vi "01 Washer HCC SM.vi"() -> ()   [LabVIEW 2011]
uses:
  HCC Data.ctl
  Washer Status Ctrl.ctl
  HCC Global Cluster Type.ctl
  <vilib>/Platform/fileVersionInfo.llb/FileVersionInformation.ctl
  GEA2 Washer Interface Ctrl.ctl
  Globals HCC.vi
panel:
  in  "Run":u32(colorbox)=6618880
  in  "Caution":u32(colorbox)=16776960
  in  "Uncofigured":u32(colorbox)=7171459
  in  "Configured":u32(colorbox)=16860
  in  "No Com":u32(colorbox)
  out "Row C":T1[](array[typedef])
  out "Init Com port message":string
  out "Row B":T1[](array[typedef])
  out "Row F":T1[](array[typedef])
  out "Row E":T1[](array[typedef])
  out "Row D":T1[](array[typedef])
  in  "Tab Control":T3(tab)=enum."View Streaming Data"
  out "Label Com Array":string[][](array[string])=[["M1", "100"], ["M3", "3"], ["M5", "5"], ["M7", "7"], ["M9", "9"], ["M11", "11"], ["M13", "13"], ["M15", "15"], ["M17", "17"], ["M19", "19"], ["M2", "2"], ["M4", "4"], ["M6", "6"], ["M8", "8"], ["M10", "10"], ["M12", "12"], ["M14", "14"], ["M16", "16"], ["M18", "18"], ["M20", "20"], ["N6", "21"], ["N7", "22"], ["N8", "23"], ["N9", "24"], ["N10", "25"], ["N11", "26"], ["N12", "27"], ["N13", "28"]]
  out "Current Filename":path
  in  "Config File":path=path "C:/Program Files/GE/Washer Hcc/HCC_Config.ini"
  out "Test Config Out":T4={"Directories"={"Com Port Config Filename"=path "D:/Work/HCC_Config.csv", "Save File Directory"=path "D:/Data", "Library Batch File"=path "c:/Data"}, "Test Information"={"Timeout"=1000, "Data Set ID"="HCC Rows A-D"}}
  in  "Timeout":i32=1000
  out "Save File Path":path=path "C:/Data"
  out "FileVersionInfo Out":T5
  out "Debug State Array":string[](array[string])
  out "Saving":errorcluster
  out "Log Coms Array":string[](array[string])
  out "Data Present":bool[](array[boolean])
  out "Partial Messages Out":cluster{"Partial Message Out":u8[]}[](array[cluster])
  in  "Select Station":string(combo)
  in  "Debug Log":string
  in  "Row Size Limits":i32[](array[numeric])=[9, 14, 19, 14, 20, 11]
  in  "Init":bool
  out "Read_ACK":bool
  out "Reading":bool
  in  "Row A":T1[](array[typedef])
  in  "Exit":bool
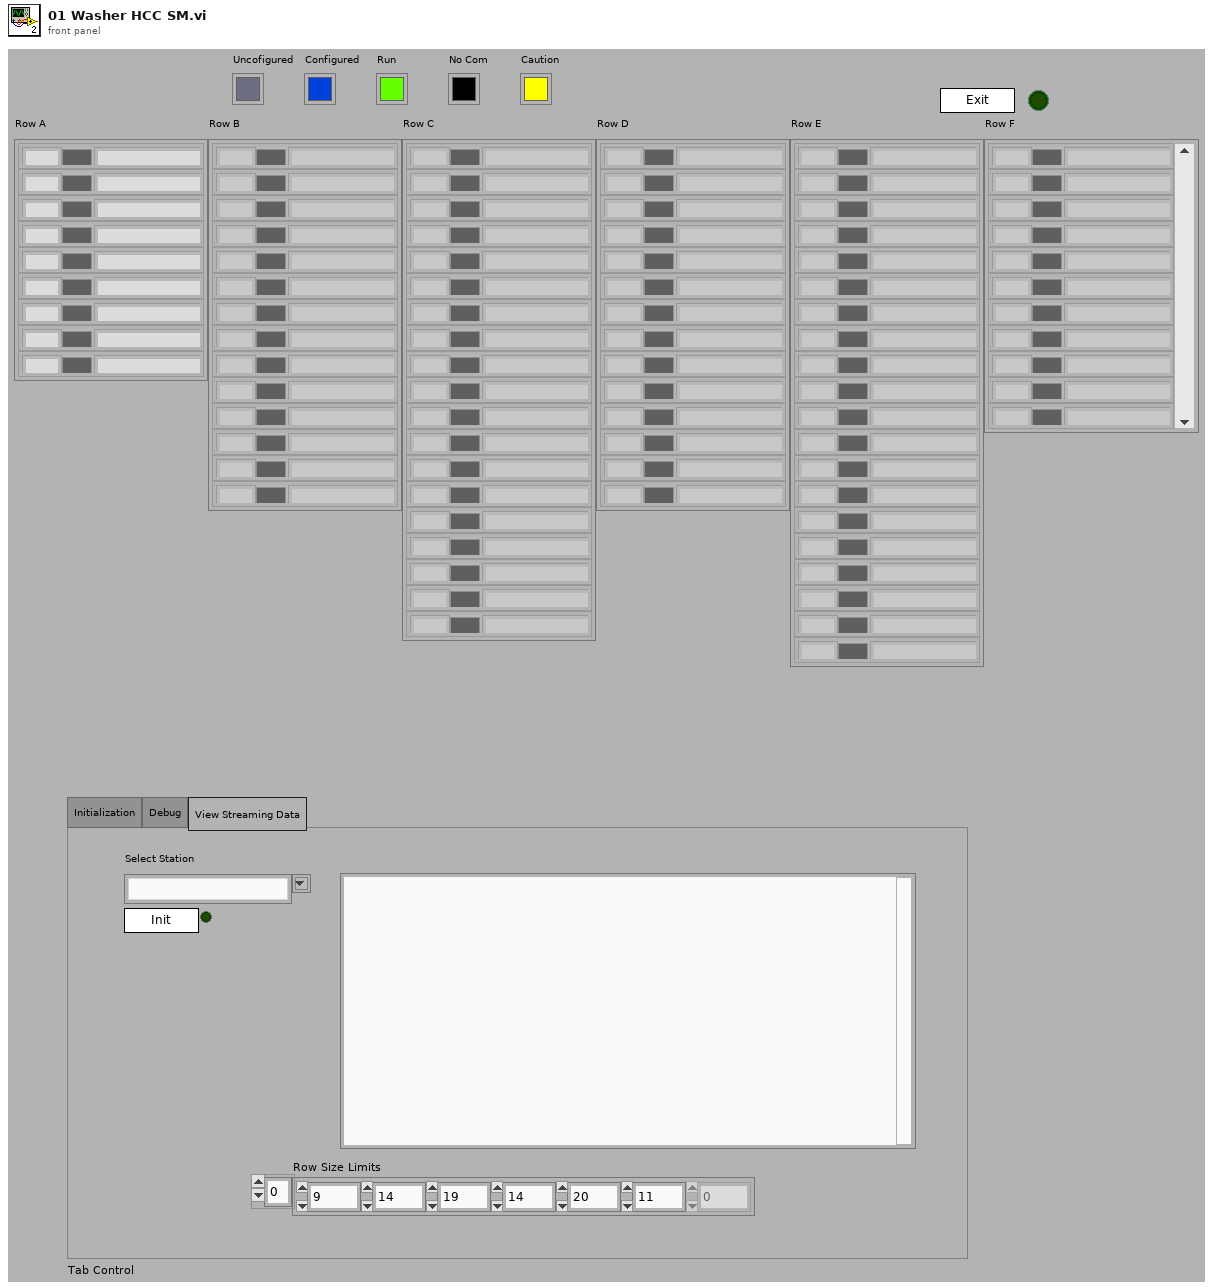
[diagram p1: front panel]
types:
  T1 = typedef "HCC Data.ctl" = cluster{"Station":string, "Color":u32, "Status":T2, "Error Time":string, "Com Err Count":u32, "Debug Log":string}
  T2 = typedef "Washer Status Ctrl.ctl" = enum16{"Running", "Err", "No Com", "No Conf"}
  T3 = enum32{"Initialization", "Debug", "View Streaming Data"}
  T4 = typedef "HCC Global Cluster Type.ctl" = cluster{"Directories":cluster{"Com Port Config Filename":path, "Save File Directory":path, "Library Batch File":path}, "Test Information":cluster{"Timeout":i32, "Data Set ID":string}}
  T5 = typedef "FileVersionInformation.ctl" = cluster{"FileVersion":string, "ProductName":string, "InternalName":string, "CompanyName":string, "LegalCopyright":string, "FileDescription":string}
  T6 = typedef "GEA2 Washer Interface Ctrl.ctl" = enum16{"Init Com Port", "SendCMD", "ReadPort", "Close Port", "Send Byte Data", "Read Continuous"}
  T7 = enum32{"invalid app kind", "Development System", "Run Time System", "Student Edition", "Embedded LabVIEW", "Evaluation", "Custom"}
  T8 = enum32{"Invalid", "Standard", "Closed", "Hidden", "Minimized", "Maximized"}
  T9 = cluster{"Core":cluster{"Current VI Reference":refnum<vi>, "Close Panel on Exit?":bool}, "Label Com Array":string[][], "Row A":T1[], "Com Array":u8[], "Save File Directory":path, "Last Hour":string, "Library Batch File":path, "Data Set ID":string}
  T10 = cluster{"Current VI Reference":refnum<vi>, "Close Panel on Exit?":bool}
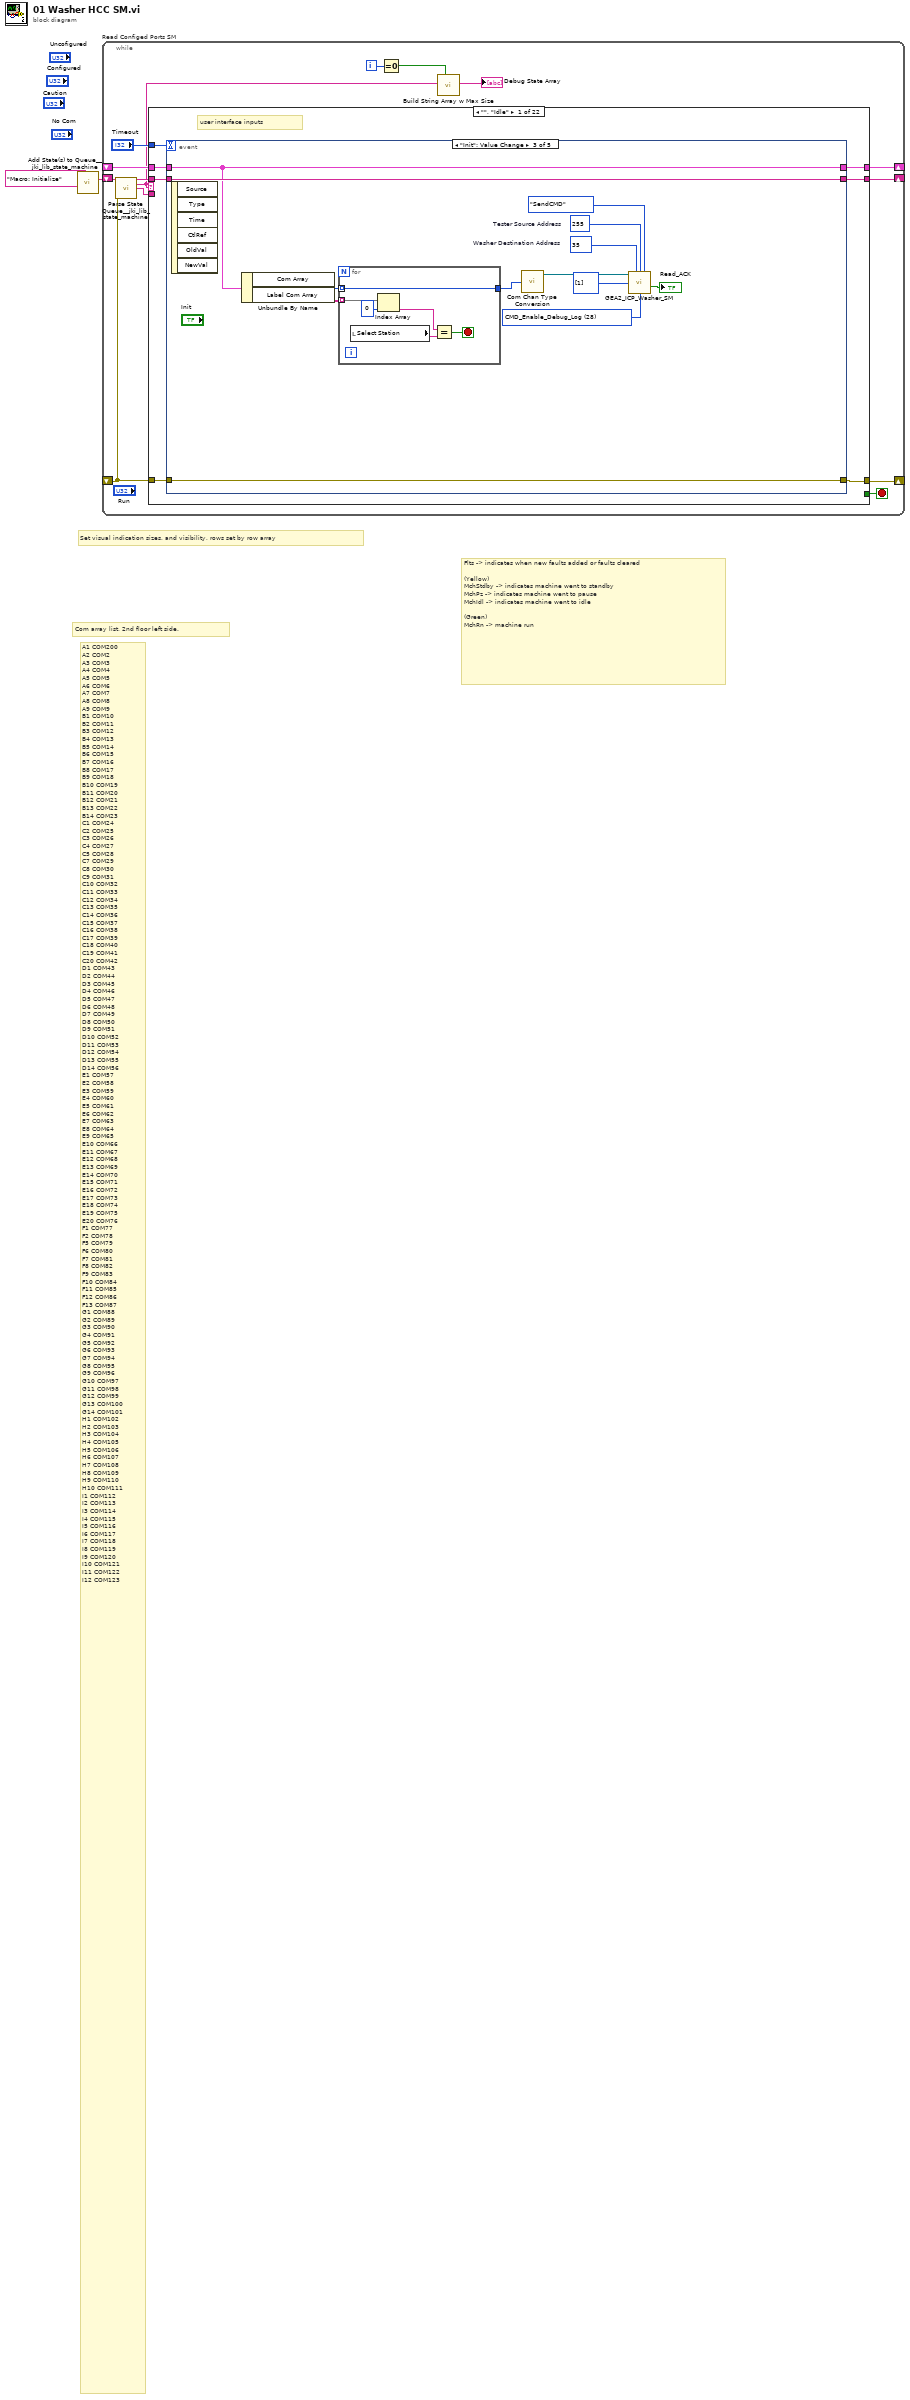
[diagram p0: block diagram]
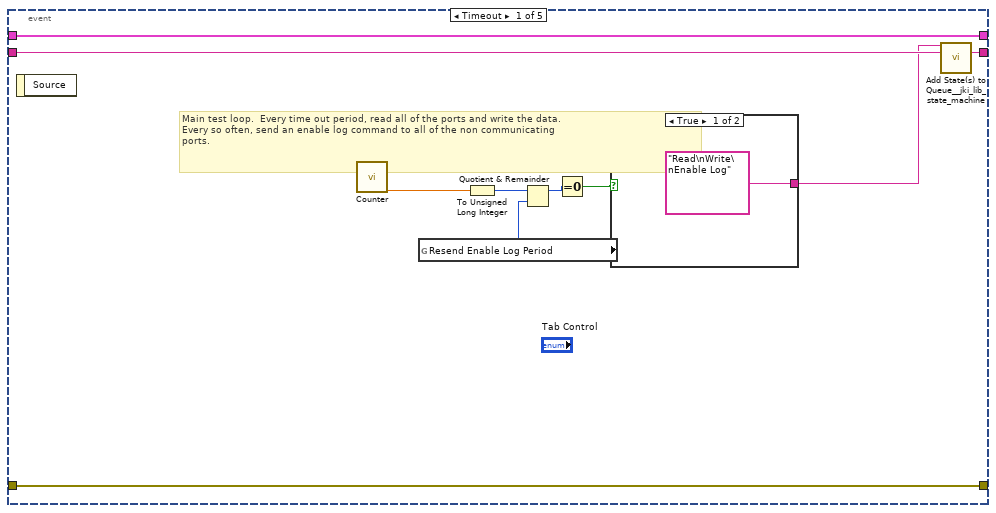
[diagram p2: hidden frame]
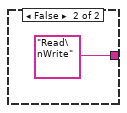
[diagram p3: hidden frame]
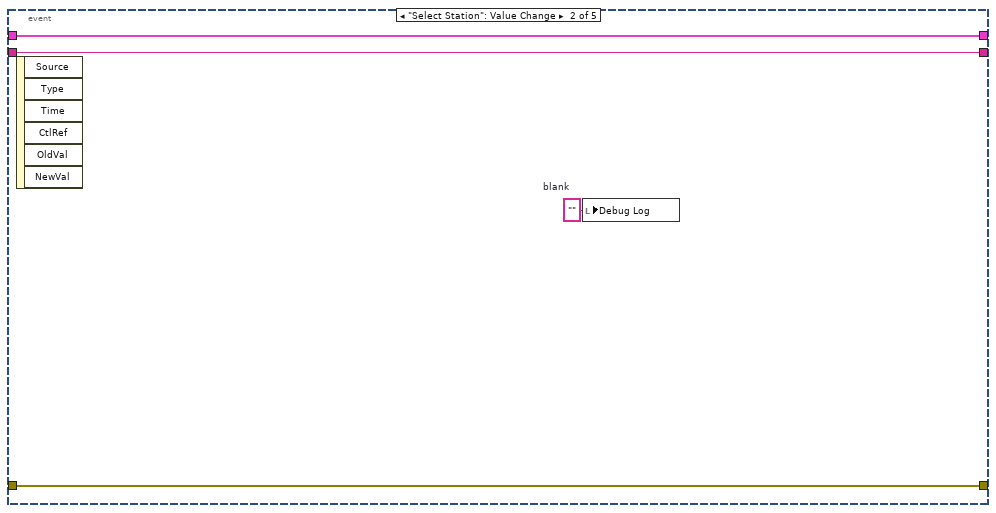
[diagram p4: hidden frame]
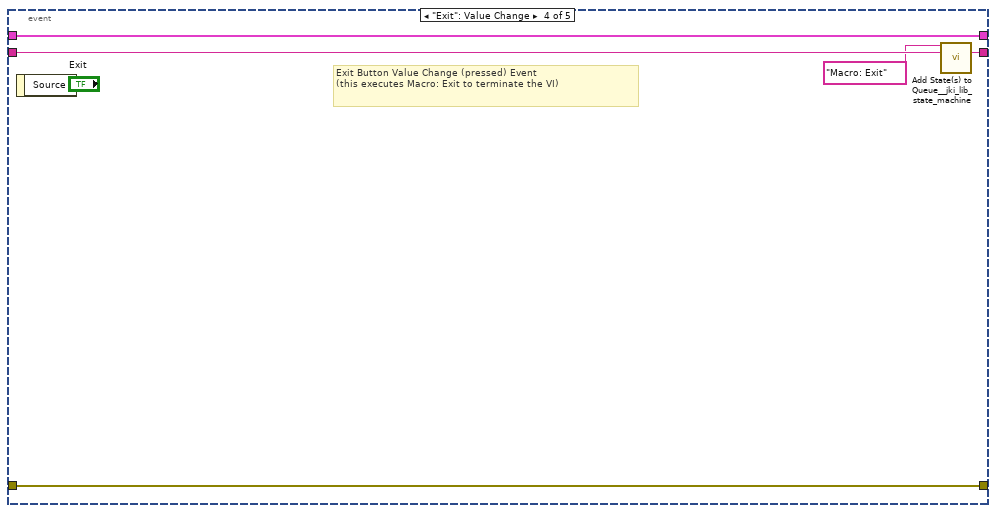
[diagram p5: hidden frame]
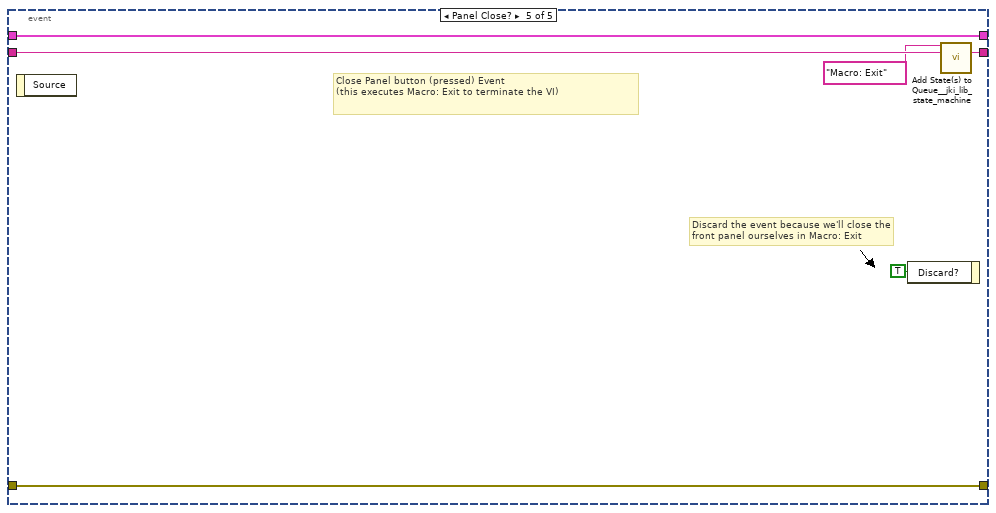
[diagram p6: hidden frame]
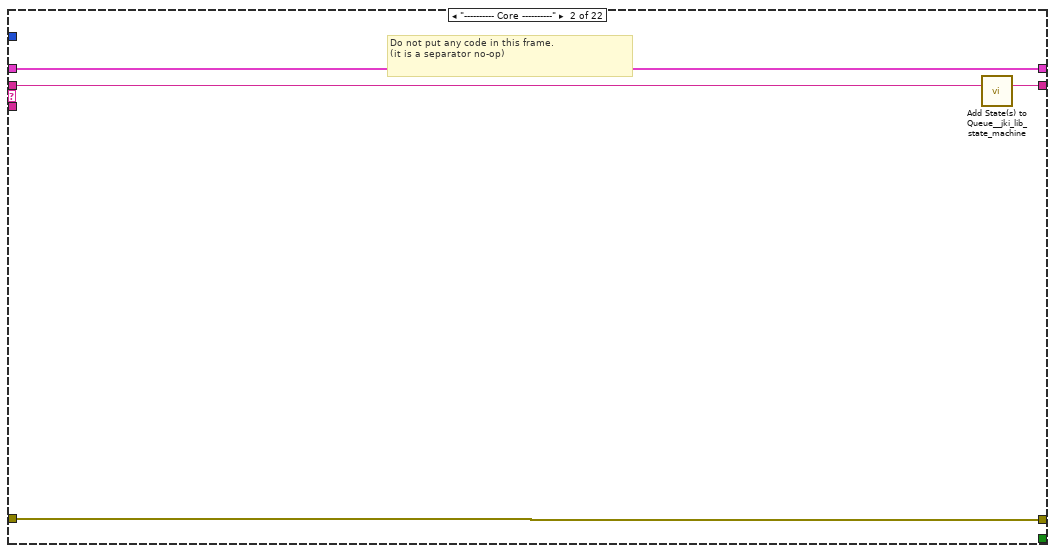
[diagram p7: hidden frame]
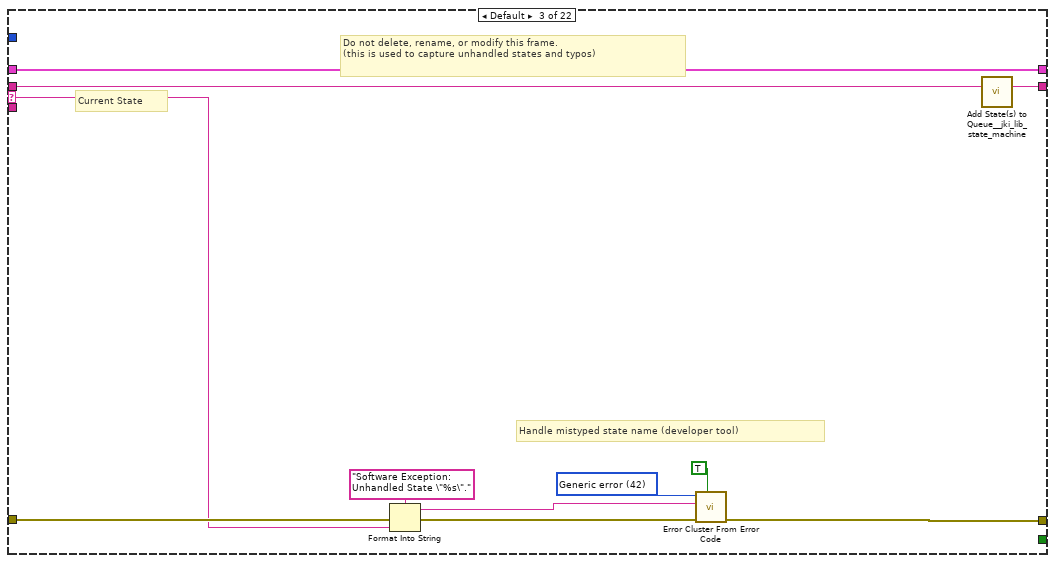
[diagram p8: hidden frame]
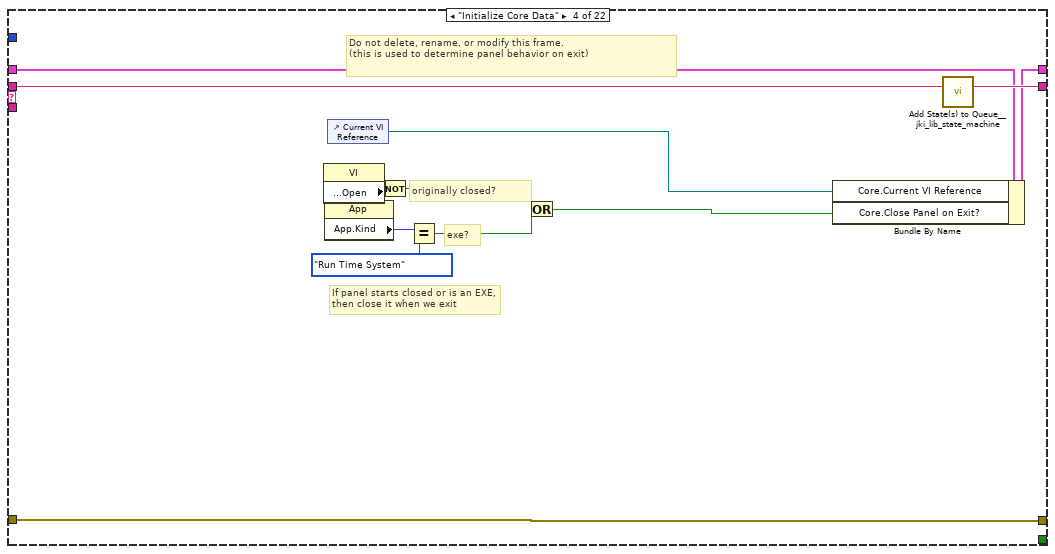
[diagram p9: hidden frame]
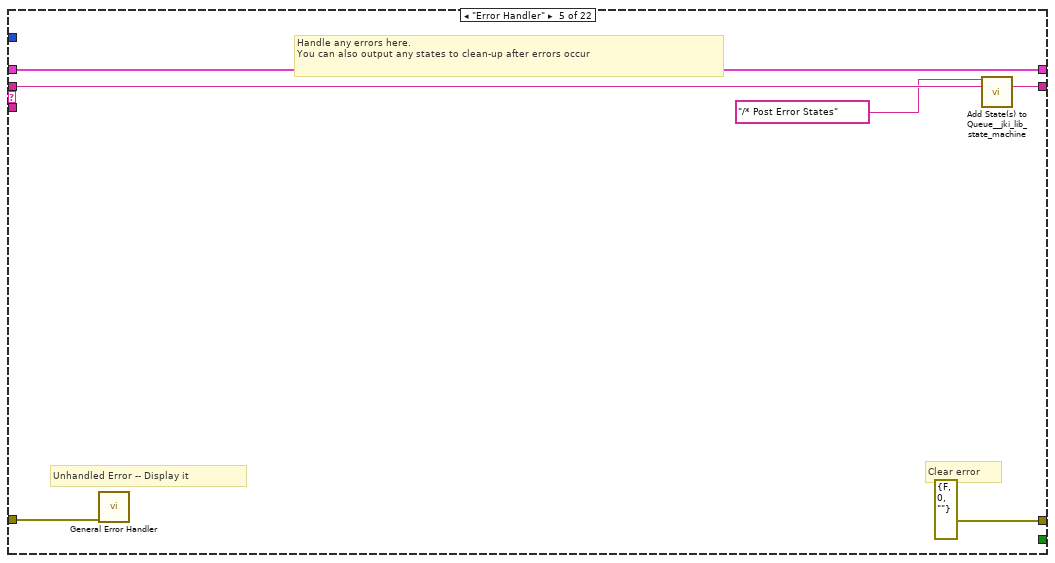
[diagram p10: hidden frame]
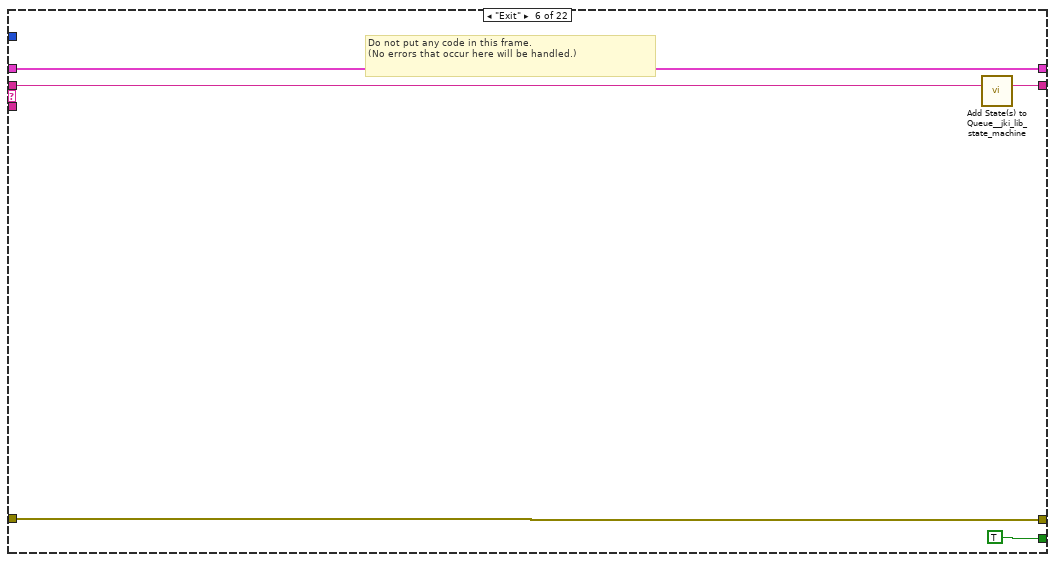
[diagram p11: hidden frame]
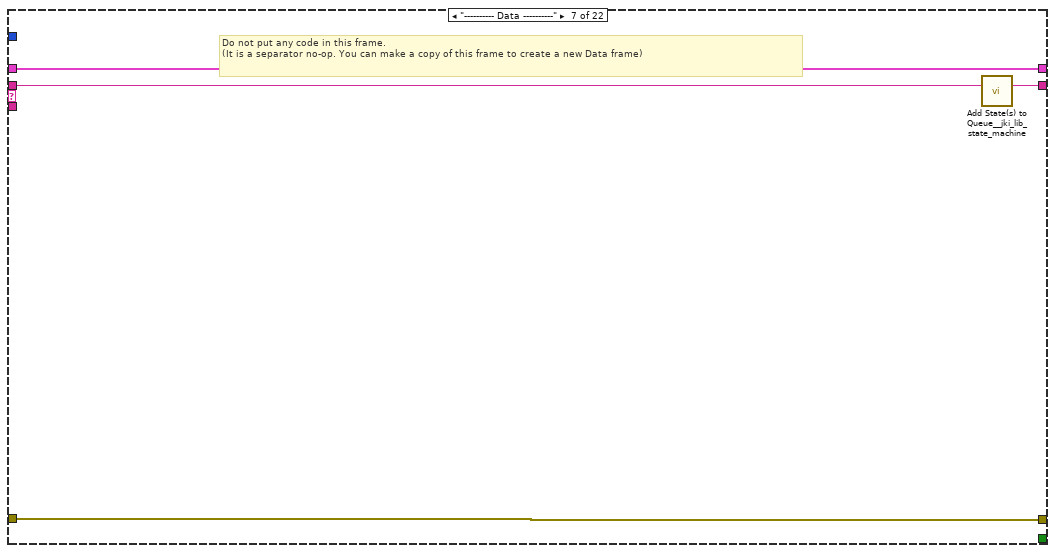
[diagram p12: hidden frame]
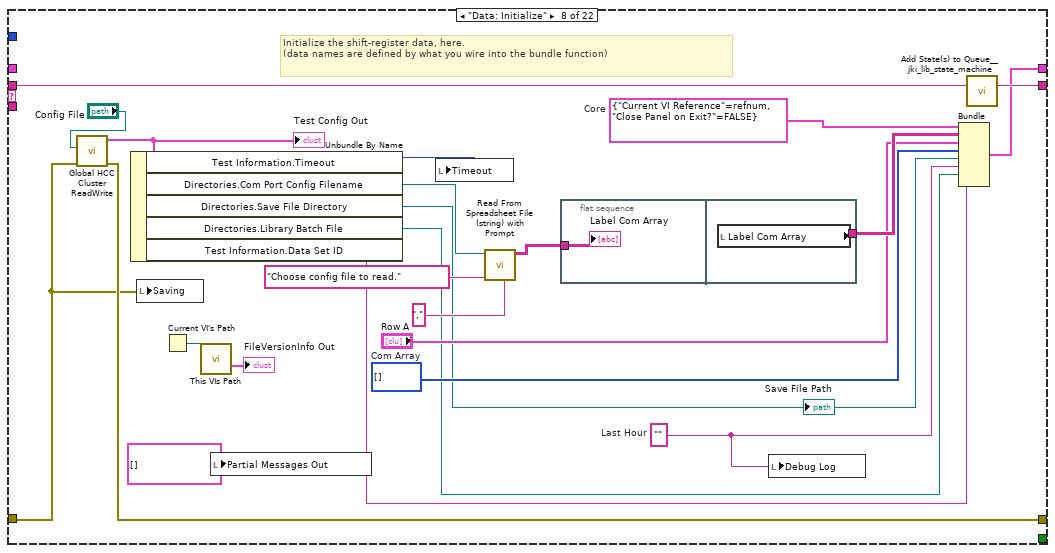
[diagram p13: hidden frame]
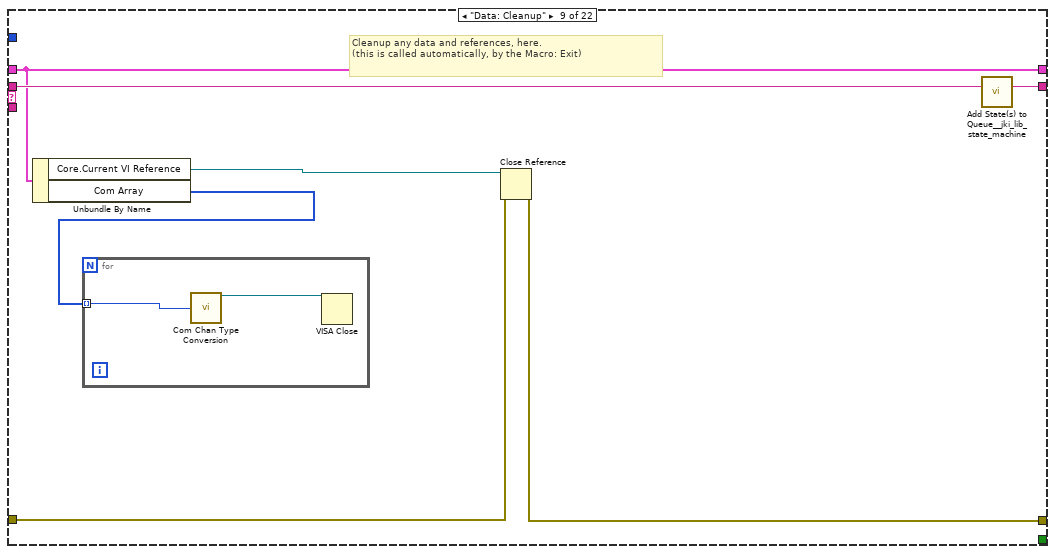
[diagram p14: hidden frame]
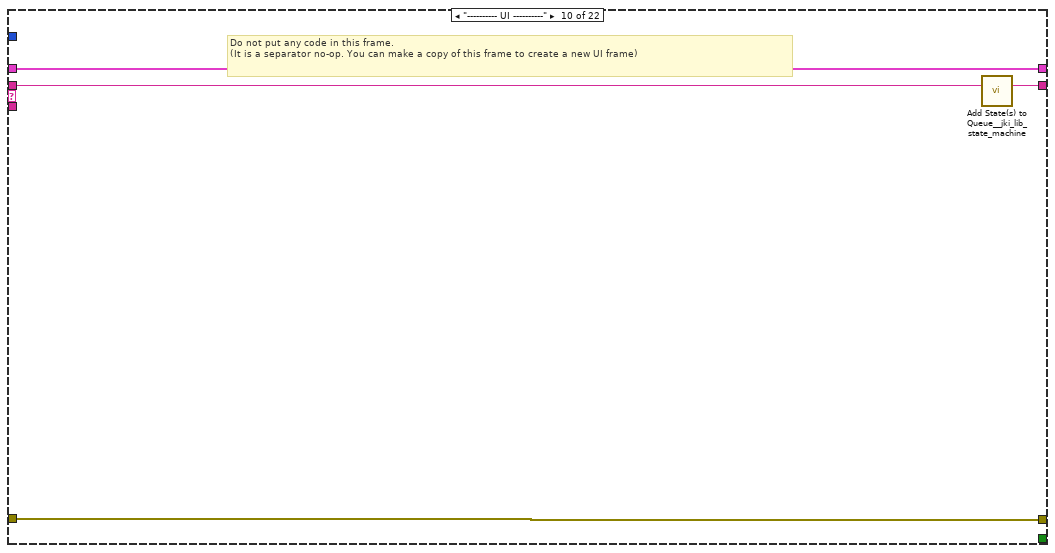
[diagram p15: hidden frame]
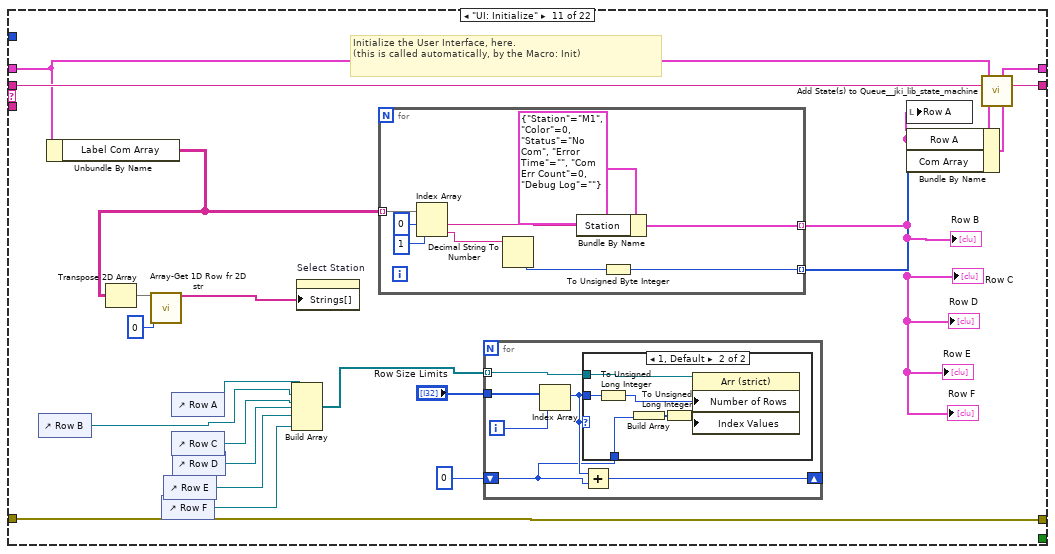
[diagram p16: hidden frame]
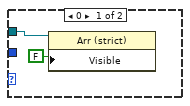
[diagram p17: hidden frame]
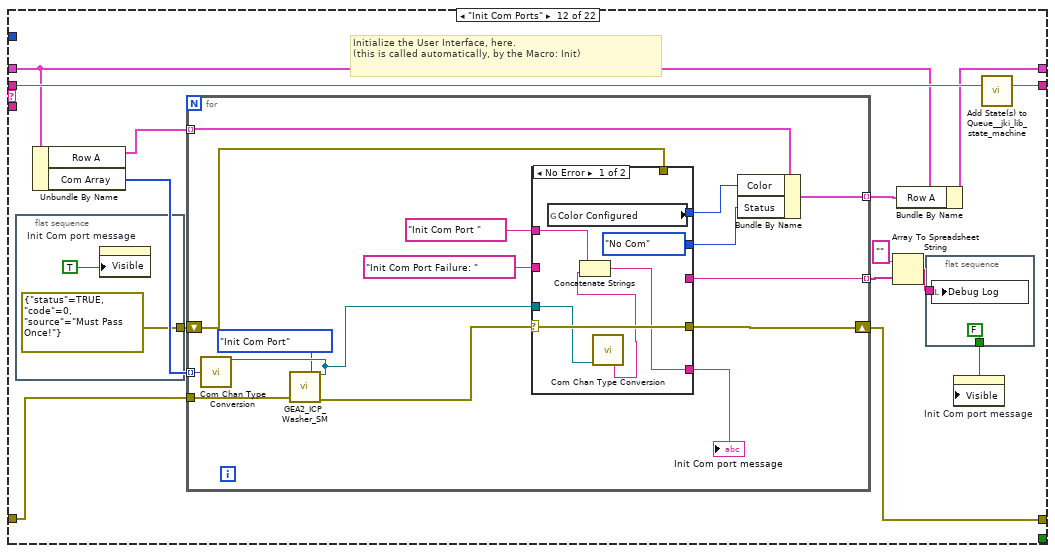
[diagram p18: hidden frame]
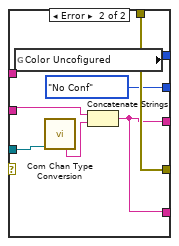
[diagram p19: hidden frame]
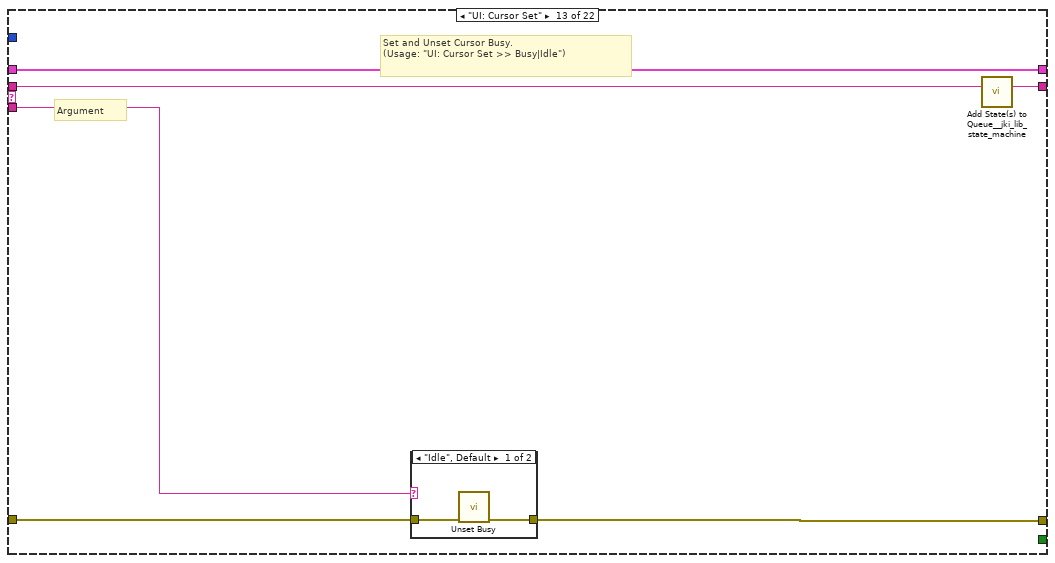
[diagram p20: hidden frame]
diagram:
  # "Com array list, 2nd floor left side."
  # "A1\tCOM200\nA2\tCOM2\nA3\tCOM3\nA4\tCOM4\nA5\tCOM5\nA6\tCOM6\nA7\tCOM7\nA8\tCOM8\nA9\tCOM9\nB1\tCOM10\nB2\tCOM11\nB3\tCOM12\nB4\tCOM13\nB5\tCOM14\nB6\tCOM15\nB7\tCOM16\nB8\tCOM17\nB9\tCOM18\nB10\tCOM19\nB11\tCOM20\nB12\tCOM21\nB13\tCOM22\nB14\tCOM23\nC1\tCOM24\nC2\tCOM25\nC3\tCOM26\nC4\tCOM27\nC5\tCOM28\nC7\tCOM29\nC8\tCOM30\nC9\tCOM31\nC10\tCOM32\nC11\tCOM33\nC12\tCOM34\nC13\tCOM35\nC14\tCOM36\nC15\tCOM37\nC16\tCOM38\nC17\tCOM39\nC18\tCOM40\nC19\tCOM41\nC20\tCOM42\nD1\tCOM43\nD2\tCOM44\nD3\tCOM45\nD4\tCOM46\nD5\tCOM47\nD6\tCOM48\nD7\tCOM49\nD8\tCOM50\nD9\tCOM51\nD10\tCOM52\nD11\tCOM53\nD12\tCOM54\nD13\tCOM55\nD14\tCOM56\nE1\tCOM57\nE2\tCOM58\nE3\tCOM59\nE4\tCOM60\nE5\tCOM61\nE6\tCOM62\nE7\tCOM63\nE8\tCOM64\nE9\tCOM65\nE10\tCOM66\nE11\tCOM67\nE12\tCOM68\nE13\tCOM69\nE14\tCOM70\nE15\tCOM71\nE16\tCOM72\nE17\tCOM73\nE18\tCOM74\nE19\tCOM75\nE20\tCOM76\nF1\tCOM77\nF2\tCOM78\nF5\tCOM79\nF6\tCOM80\nF7\tCOM81\nF8\tCOM82\nF9\tCOM83\nF10\tCOM84\nF11\tCOM85\nF12\tCOM86\nF13\tCOM87\nG1\tCOM88\nG2\tCOM89\nG3\tCOM90\nG4\tCOM91\nG5\tCOM92\nG6\tCOM93\nG7\tCOM94\nG8\tCOM95\nG9\tCOM96\nG10\tCOM97\nG11\tCOM98\nG12\tCOM99\nG13\tCOM100\nG14\tCOM101\nH1\tCOM102\nH2\tCOM103\nH3\tCOM104\nH4\tCOM105\nH5\tCOM106\nH6\tCOM107\nH7\tCOM108\nH8\tCOM109\nH9\tCOM110\nH10\tCOM111\nI1\tCOM112\nI2\tCOM113\nI3\tCOM114\nI4\tCOM115\nI5\tCOM116\nI6\tCOM117\nI7\tCOM118\nI8\tCOM119\nI9\tCOM120\nI10\tCOM121\nI11\tCOM122\nI12\tCOM123"
  # "Set visual indication sizes, and visibility, rows set by row array"
  # "Flts -> indicates when new faults added or faults cleared\n\n(Yellow)\nMchStdby -> indicates machine went to standby\nMchPz -> indicates machine went to pause\nMchIdl -> indicates machine went to idle \n\n(Green)\nMchRn -> machine run"
  n1 = call <vilib>:"Add State(s) to Queue__jki_lib_state_machine.vi"("State(s) in (\"\")"="Macro: Initialize") -> ("States Out"=w2:string)  [unwired: 14 in]
  n2 = while "Read Configed Ports SM" {
    shift-right: [w10] -> _
    shift-left: _ -> [w9]
    shift-right: [w13] -> _
    shift-left: _ -> [w7]
    shift-right: [w12] -> _
    shift-left: w2 -> [w14]
    i -> [w3]
    stop <- w11 stop-if-true
    n3 = call <vilib>:"Parse State Queue__jki_lib_state_machine.vi"("State Queue"=w14, "Error In (no error)"=w7) -> ("Remaining States"=w16:string, "Current State"=w6:string, "Arguments"=w15:string)  [unwired: 11 in]
    n4 = case shown="\"\", \"Idle\"" w6 {
      selector: w6 -> [_ _ w74 _ _ _ _ _ _ _ _ _ _ _ _ _ _ _ _ _ _ _]
      tunnel: w16 -> [w23 w73 w78 w96 w102 w107 w111 w134 w143 w149 w169 w206 w245 w256 w282 w287 w297 w301 w314 w331 w369 w382]
      tunnel: w15 -> [_ _ _ _ _ _ _ _ _ _ _ _ w240 w250 _ _ _ _ _ _ _ _]
      tunnel: w9 -> [w21 w70 w76 w87 w99 w105 w108 _ w138 w146 w166 w198 w243 w252 w279 w284 w294 w298 w310 w328 w367 w378]
      tunnel: [w20 w71 w80 w93 errorcluster {"status"=FALSE, "code"=0, "source"=""} ("error out") w104 w109 w118 w139 w147 w167 w202 w241 w253 w280 w285 w295 w299 w312 w329 w357 w379] -> w13
      tunnel: w7 -> [w19 w71 w79 w93 w98 w104 w109 w112 w140 w147 w167 w203 w242 w254 w280 w285 w295 w299 w312 w329 w358 w380]
      tunnel: [w22 w72 w77 w95 w101 w106 w110 w133 w142 w148 w168 w205 w244 w255 w281 w286 w296 w300 w313 w330 w368 w381] -> w12
      tunnel: [_ _ _ _ _ TRUE _ _ _ _ _ _ _ _ _ _ _ _ _ _ _ _] -> w11
      tunnel: [w18 w70 w76 w94 w99 w105 w108 w132 w138 w146 w165 w197 w243 w252 w279 w284 w294 w298 w309 w328 w366 w378] -> w10
      tunnel: "Timeout" -> [w17 _ _ _ _ _ _ _ _ _ _ _ _ _ _ _ _ _ _ _ _ _]
      frame "", "Idle" {
        # "user interface inputs"
        n5 = event shown="[2] \"Init\": Value Change" {
          selector: _ -> [_ _ _ _ _]
          dyn-events: _ -> [_ _ _ _ _]
          timeout: w17 -> [_ _ _ _ _]
          tunnel: w23 -> [w33 w38 w52 w63 w69]
          tunnel: [w32 w38 w52 w62 w68] -> w22
          tunnel: w21 -> [w30 w37 w46 w60 w66]
          tunnel: [w31 w36 w51 w61 w67] -> w20
          tunnel: w19 -> [w31 w36 w51 w61 w67]
          tunnel: [w30 w37 w46 w60 w66] -> w18
          event Timeout {
            # "Main test loop.  Every time out period, read all of the ports and write the data.\nEvery so often, send an enable log command to all of the non communicating\nports."
            n6 = event-data() -> ()  [unwired: 1 in, 1 out]
            n7 = call "Counter.vi"() -> ("Count"=w28:dbl)  [unwired: 11 in]
            n8 = global read "Globals HCC.vi" "Resend Enable Log Period"() -> (w27:u32)
            n9 = To Unsigned Long Integer(number=w28) -> (unsigned 32bit integer=w24:u32)
            n10 = Quotient & Remainder(x=w24, y=w27) -> (x-y*floor(x/y)=w26:u32)  [unwired: 1 out]
            n11 = Equal To 0?(x=w26) -> (x = 0?=w25:bool)
            n12 = case shown="True" w25 {
              tunnel: ["Read\nWrite\nEnable Log" ("State(s) in Front (\"\")") "Read\nWrite" ("State(s) in Front (\"\")")] -> w29
              frame True {
              }
              frame False {
              }
            }
            n13 = call <vilib>:"Add State(s) to Queue__jki_lib_state_machine.vi"("State(s) in Front (\"\")"=w29, "State(s) in (\"\")"=w33) -> ("States Out"=w32:string)  [unwired: 13 in]
          }
          event "Select Station": Value Change {
            w39 = ""  # blank
            n14 = event-data() -> ()  [unwired: 1 in, 6 out]
            n15 = local write "Debug Log"(w39) -> ()
          }
          event "Init": Value Change {
            w41 = u8 28 items=["CMD_Entry_Command", "CMD_Load_Control", "RQST_Input_Status", "CMD_LED_Control", "RQST_Encoder_Position_Status", "RQST_A2D_Status", "RQST_Switch_States_Status", "CMD_Buzzer_Control", "CMD_Shift_to_Spin", "CMD_Shift_to_Agitate", "RQST_Mode_Shift_Complete_Status", "CMD_Control_Inverter", "CMD_Spin_Action", "CMD_Agitate_Action", "RQST_Total_Switch_Status", "RQST_Total_Encoder_Status", "CMD_Test_Eeprom", "RQST_Eeprom_Test_Status", "CMD_Power_Mode", "RQST_Error_Status", "RQST_Get_Version", "CMD_Set_Personality", "RQST_Get_Personality", "CMD_Serial_Number", "RQST_Serial_Number_Status", "CMD_Model_Number", "RQST_Model_Number_Status", "CMD_Enter_Boot_Loader", "CMD_Enable_Debug_Log"] ("Command")
            w49 = u8 255  # Tester Source Address
            w50 = u8 35  # Washer Destination Address
            n16 = event-data() -> ()  [unwired: 1 in, 6 out]
            n17 = Unbundle By Name(w46) -> ("Com Array"=w48:u8[], "Label Com Array"=w47:string[][])
            n18 = for {
              tunnel: w47 -> [w58] mode=indexing
              tunnel: w48 -> [w53] mode=indexing
              tunnel: [w53] -> w45
              stop <- w55 stop-if-true
              n19 = local read "Select Station"() -> (w54:string)
              n20 = Index Array(array=w58, index=0) -> (element=w56:string)
              n21 = Equal?(x=w56, y=w54) -> (x = y?=w55:bool)
            }
            n22 = call "Com Chan Type Conversion.vi"("Com Chan"=w45) -> ("VISA resource name"=w44:refnum<visa-resource-name>)  [unwired: 11 in, 3 out]
            n23 = call "GEA2_ICP_Washer_SM.vi"("ComPort"=w44, "Destination Address"=w50, "Source Address"=w49, "Mode"=GEA2_Washer_Interface_Ctrl."SendCMD", "Byte Data"=u8[] [1], "Command"=w41) -> ("WriteOK"=→"Read_ACK":bool)  [unwired: 6 in, 3 out]
          }
          event "Exit": Value Change {
            # "Exit Button Value Change (pressed) Event\n(this executes Macro: Exit to terminate the VI)"
            n24 = event-data() -> ()  [unwired: 1 in, 1 out]
            n25 = call <vilib>:"Add State(s) to Queue__jki_lib_state_machine.vi"("State(s) in Front (\"\")"="Macro: Exit", "State(s) in (\"\")"=w63) -> ("States Out"=w62:string)  [unwired: 13 in]
          }
          event Panel Close? {
            # "Discard the event because we'll close the front panel ourselves in Macro: Exit"
            # "Close Panel button (pressed) Event\n(this executes Macro: Exit to terminate the VI)"
            n26 = event-data() -> ()  [unwired: 1 in, 1 out]
            n27 = event-data("Discard?"=TRUE) -> ()  [unwired: 1 in, 1 out]
            n28 = call <vilib>:"Add State(s) to Queue__jki_lib_state_machine.vi"("State(s) in Front (\"\")"="Macro: Exit", "State(s) in (\"\")"=w69) -> ("States Out"=w68:string)  [unwired: 13 in]
          }
        }
      }
      frame "---------- Core ----------" {
        # "Do not put any code in this frame.\n(it is a separator no-op)"
        n29 = call <vilib>:"Add State(s) to Queue__jki_lib_state_machine.vi"("State(s) in (\"\")"=w73) -> ("States Out"=w72:string)  [unwired: 14 in]
      }
      frame Default {
        w83 = 42 items=["No error", "Argument error", "Memory is full", "Out of zone", "End of file", "File already open", "Generic file I/O error", "File not found", "File permission error", "Disk is full", "Duplicate path", "Too many files open", "System feature not enabled", "Resource file not found", "Cannot add resource", "Resource not found", "Image not found", "Image memory error", "Pen does not exist", "Config type invalid", "Config token not found", "Config parse error", "Config memory error", "Bad external code format", "Bad external code offset", "External code not present", "Null window", "Destroy window error", "Null menu", "Print aborted", "Bad print record", "Print driver error", "Windows error during printing", "Memory error during printing", "Print dialog error", "Generic print error", "Invalid device refnum", "Device not found", "Device parameter error", "Device unit error", "Cannot open device", "Device call aborted", "Generic error", "Cancelled by user", "Object ID too low", "Object ID too high", "Object not in heap", "Unknown heap", "Unknown object (invalid DefProc)", "Unknown object (DefProc not in table)", "Message out of range", "Invalid (null) method", "Unknown message", "Manager call not supported", "Bad address", "Network operation in progress", "Network operation timed out", "Connection is busy", "Network attribute not supported", "Network error", "Address in use", "System out of memory", "Connection aborted", "Connection refused", "Not connected", "Already connected", "Connection closed", "Initialization error (interapplication manager)", "Bad occurrence", "Wait on unbound occurrence handler", "Occurrence queue overflow", "Datalog type conflict", "Unused", "Unrecognized type (interapplication manager)", "Memory corrupt", "Failed to make temporary DLL", "Old CIN version", "Drag socket not found", "Failed to load drop-object", "Failed to register OLE object", "Failed to release OLE object", "Format specifier type mismatch", "Unknown format specifier", "Too few format specifiers", "Too many format specifiers", "Scan failed", "Newer CIN version", "Error converting to variant", "Runtime menu error", "Password tampered", "Variant attribute not found", "Incompatible variant data type", "Event data is not available", "Event Store is not present", "Occurrence is not found", "Event Queue is not created", "Event info is not available", "Refnum passed is NULL", "Error retrieving Class GUID", "Error retrieving CoClass GUID", "Error retrieving TypeLib GUID.", "Bad built application magic bytes.", "Specific driver is different from the specific driver associated with the Logical Name.", "There is no session opened to the class driver.", "Max Error", "MAX - Error with config objects", "MAX - Error loading configuration", "MAX - Group not supported"]
        # "Current State"
        # "Do not delete, rename, or modify this frame.\n(this is used to capture unhandled states and typos)"
        # "Handle mistyped state name (developer tool)"
        n30 = Format Into String(format string="Software Exception: Unhandled State \"%s\"." ("message"), error in=w79, w74) -> (resulting string=w82:string, error out=w81:errorcluster)  [unwired: 1 in]
        n31 = call <vilib>:"Error Cluster From Error Code.vi"("show call chain? (False)"=TRUE, "error in (no error)"=w81, "error message (\"\")"=w82, "error code (0)"=w83) -> ("error out"=w80:errorcluster)  [unwired: 5 in]
        n32 = call <vilib>:"Add State(s) to Queue__jki_lib_state_machine.vi"("State(s) in (\"\")"=w78) -> ("States Out"=w77:string)  [unwired: 14 in]
      }
      frame "Initialize Core Data" {
        # "Do not delete, rename, or modify this frame.\n(this is used to determine panel behavior on exit)"
        # "originally closed?"
        # "exe?"
        # "If panel starts closed or is an EXE, then close it when we exit"
        n33 = property class="VI"() -> ("Front Panel.Open"=w92:bool)  [unwired: 2 in, 2 out]
        n34 = property class="App"() -> ("App.Kind"=w91:T7)  [unwired: 2 in, 2 out]
        n35 = control-ref of="Current VI Reference"() -> (w85:refnum<vi>)
        n36 = Not(x=w92) -> (.not. x?=w89:bool)
        n37 = Equal?(x=w91, y=T7."Run Time System" ("Application:Kind")) -> (x = y?=w88:bool)
        n38 = Or(x=w89, y=w88) -> (x .or. y?=w86:bool)
        n39 = Bundle By Name(cluster=w87, "Core.Current VI Reference"=w85, "Core.Close Panel on Exit?"=w86) -> (w94:T9)
        n40 = call <vilib>:"Add State(s) to Queue__jki_lib_state_machine.vi"("State(s) in (\"\")"=w96) -> ("States Out"=w95:string)  [unwired: 14 in]
      }
      frame "Error Handler" {
        # "Unhandled Error -- Display it"
        # "Handle any errors here.\nYou can also output any states to clean-up after errors occur"
        # "Clear error"
        n41 = call <vilib>:"General Error Handler.vi"("error in (no error)"=w98) -> ()  [unwired: 10 in, 5 out]
        n42 = call <vilib>:"Add State(s) to Queue__jki_lib_state_machine.vi"("State(s) in Front (\"\")"="/* Post Error States", "State(s) in (\"\")"=w102) -> ("States Out"=w101:string)  [unwired: 13 in]
      }
      frame "Exit" {
        # "Do not put any code in this frame.\n(No errors that occur here will be handled.)"
        n43 = call <vilib>:"Add State(s) to Queue__jki_lib_state_machine.vi"("State(s) in (\"\")"=w107) -> ("States Out"=w106:string)  [unwired: 14 in]
      }
      frame "---------- Data ----------" {
        # "Do not put any code in this frame.\n(It is a separator no-op. You can make a copy of this frame to create a new Data frame)"
        n44 = call <vilib>:"Add State(s) to Queue__jki_lib_state_machine.vi"("State(s) in (\"\")"=w111) -> ("States Out"=w110:string)  [unwired: 14 in]
      }
      frame "Data: Initialize" {
        w124 = ""  # Last Hour
        w126 = u8[] []  # Com Array
        w131 = T10 {"Current VI Reference"=refnum, "Close Panel on Exit?"=FALSE}  # Core
        # "Initialize the shift-register data, here.\n(data names are defined by what you wire into the bundle function)"
        n45 = call "Global HCC Cluster ReadWrite.vi"("error in (no error)"=w112, "configuration file path"="Config File") -> ("error out"=w118:errorcluster, "Test Config Out"=w122:T4)  [unwired: 8 in]
        "Test Config Out" <- w122
        n46 = Unbundle By Name(w122) -> ("Test Information.Timeout"=w119:i32, "Directories.Com Port Config Filename"=w121:path, "Directories.Save File Directory"=w117:path, "Directories.Library Batch File"=w120:path, "Test Information.Data Set ID"=w116:string)
        "Save File Path" <- w117
        n47 = local write "Saving"(w112) -> ()
        n48 = Current VI's Path() -> (path=w114:path)
        n49 = call "This VIs Path.vi"("path"=w114) -> ("FileVersionInfo Out"=→"FileVersionInfo Out":T5)  [unwired: 10 in, 4 out]
        n50 = local write "Partial Messages Out"(cluster{"Partial Message Out":u8[]}[] [] ("Partial Messages Out")) -> ()
        n51 = local write "Timeout"(w119) -> ()
        n52 = call "Read From Spreadsheet File (string) with Prompt.vi"("delimiter (\\t)"="," ("delimiter (\\t)"), "prompt"="Choose config file to read.", "file path (dialog if empty)"=w121) -> ("all rows"=w129:string[][])  [unwired: 4 in, 4 out]
        n53 = flat-sequence {
          tunnel: w129 -> [w135]
          tunnel: [w136] -> w128
          frame #0 {
            "Label Com Array" <- w135
          }
          frame #1 {
            n54 = local read "Label Com Array"() -> (w136:string[][])
          }
        }
        n55 = local write "Debug Log"(w124) -> ()
        n56 = Bundle("Core"=w131, "Label Com Array"=w128, "Row A"="Row A", "Com Array"=w126, "Save File Directory"=w117, "Last Hour"=w124, "Library Batch File"=w120, "Data Set ID"=w116) -> (w132:T9)  [unwired: 1 in]
        n57 = call <vilib>:"Add State(s) to Queue__jki_lib_state_machine.vi"("State(s) in (\"\")"=w134) -> ("States Out"=w133:string)  [unwired: 14 in]
      }
      frame "Data: Cleanup" {
        # "Cleanup any data and references, here.\n(this is called automatically, by the Macro: Exit)"
        n58 = Unbundle By Name(w138) -> ("Core.Current VI Reference"=w141:refnum<vi>, "Com Array"=w137:u8[])
        n59 = for {
          tunnel: w137 -> [w145] mode=indexing
          n60 = call "Com Chan Type Conversion.vi"("Com Chan"=w145) -> ("VISA resource name"=w144:refnum<visa-resource-name>)  [unwired: 11 in, 3 out]
          n61 = VISA Close(VISA resource name=w144) -> ()  [unwired: 1 in, 1 out]
        }
        n62 = Close Reference(reference=w141, error in (no error)=w140) -> (error out=w139:errorcluster)
        n63 = call <vilib>:"Add State(s) to Queue__jki_lib_state_machine.vi"("State(s) in (\"\")"=w143) -> ("States Out"=w142:string)  [unwired: 14 in]
      }
      frame "---------- UI ----------" {
        # "Do not put any code in this frame.\n(It is a separator no-op. You can make a copy of this frame to create a new UI frame)"
        n64 = call <vilib>:"Add State(s) to Queue__jki_lib_state_machine.vi"("State(s) in (\"\")"=w149) -> ("States Out"=w148:string)  [unwired: 14 in]
      }
      frame "UI: Initialize" {
        # "Initialize the User Interface, here.\n(this is called automatically, by the Macro: Init)"
        n65 = control-ref of="Row B"() -> (w150:refnum<vi>)
        n66 = Unbundle By Name(w166) -> ("Label Com Array"=w162:string[][])
        n67 = Transpose 2D Array(2D array=w162) -> (transposed array=w163:string[][])
        n68 = call "Array-Get 1D Row fr 2D str.vi"("all rows"=w163, "row index"=0) -> ("row"=w160:string[])  [unwired: 13 in]
        n69 = control-ref of="Row F"() -> (w152:refnum<vi>)
        n70 = control-ref of="Row E"() -> (w155:refnum<vi>)
        n71 = control-ref of="Row A"() -> (w158:refnum<vi>)
        n72 = control-ref of="Row C"() -> (w157:refnum<vi>)
        n73 = control-ref of="Row D"() -> (w156:refnum<vi>)
        n74 = Build Array(w158, w150, w157, w156, w155, w152) -> (w154:refnum<vi>[])
        n75 = property on="Select Station" class="CmbBox"("Strings[]"=w160) -> ()  [unwired: 2 in, 2 out]
        n76 = for {
          tunnel: w162 -> [w192] mode=indexing
          tunnel: [w184] -> w164 mode=indexing
          tunnel: [w186] -> w151 mode=indexing
          n77 = Index Array(array=w192, index #1=0 ("index"), index #2=1 ("index")) -> (element #1=w188:string, element #2=w187:string)
          n78 = Decimal String To Number(string=w187) -> (number=w185:i32)  [unwired: 2 in, 1 out]
          n79 = Bundle By Name(cluster=T1 {"Station"="M1", "Color"=0, "Status"=enum."No Com", "Error Time"="", "Com Err Count"=0, "Debug Log"=""} ("Location:IND,Status,Message,No Com Count, Cycle Count"), "Station"=w188) -> (w186:T1)
          n80 = To Unsigned Byte Integer(number=w185) -> (unsigned 8bit integer=w184:u8)
        }
        "Row D" <- w151
        "Row E" <- w151
        "Row C" <- w151
        "Row F" <- w151
        "Row B" <- w151
        n81 = for {
          tunnel: w154 -> [w175] mode=indexing
          tunnel: "Row Size Limits" -> [w174]
          shift-right: [w171] -> _
          shift-left: 0 -> [w170]
          i -> [w173]
          n82 = Index Array(array=w174, index=w173) -> (element=w172:i32)
          n83 = case shown="1, Default" w172 {
            tunnel: w175 -> [w177 w183]
            tunnel: w172 -> [_ w182]
            tunnel: w170 -> [_ w178]
            frame 0 {
              n84 = property class="Arr (strict)"(reference=w177, "Visible"=FALSE) -> ()  [unwired: 1 in, 2 out]
            }
            frame 1, Default {
              n85 = To Unsigned Long Integer(number=w182) -> (unsigned 32bit integer=w181:u32)
              n86 = Build Array(w178) -> (w180:i32[])
              n87 = To Unsigned Long Integer(number=w180) -> (unsigned 32bit integer=w179:u32[])
              n88 = property class="Arr (strict)"(reference=w183, "Number of Rows"=w181, "Index Values"=w179) -> ()  [unwired: 1 in, 2 out]
            }
          }
          n89 = Add(x=w172, y=w170) -> (x+y=w171:i32)
        }
        n90 = local write "Row A"(w151) -> ()
        n91 = Bundle By Name(cluster=w166, "Row A"=w151, "Com Array"=w164) -> (w165:T9)
        n92 = call <vilib>:"Add State(s) to Queue__jki_lib_state_machine.vi"("State(s) in (\"\")"=w169) -> ("States Out"=w168:string)  [unwired: 14 in]
      }
      frame "Init Com Ports" {
        # "Initialize the User Interface, here.\n(this is called automatically, by the Macro: Init)"
        n93 = flat-sequence {
          tunnel: [errorcluster {"status"=TRUE, "code"=0, "source"="Must Pass Once!"} ("error IO")] -> w201
          frame #0 {
            n94 = property on="Init Com port message" class="Str"("Visible"=TRUE) -> ()  [unwired: 2 in, 2 out]
          }
        }
        n95 = Unbundle By Name(w198) -> ("Row A"=w200:T1[], "Com Array"=w204:u8[])
        n96 = for {
          tunnel: w204 -> [w224] mode=indexing
          tunnel: w203 -> [w225]
          shift-right: [w220] -> w202
          shift-left: w201 -> [w219]
          tunnel: w200 -> [w218] mode=indexing
          tunnel: [w216] -> w199 mode=indexing
          tunnel: [w215] -> w196 mode=indexing
          n97 = call "Com Chan Type Conversion.vi"("Com Chan"=w224) -> ("VISA resource name"=w223:refnum<visa-resource-name>)  [unwired: 11 in, 3 out]
          n98 = call "GEA2_ICP_Washer_SM.vi"("ComPort"=w223, "Mode"=GEA2_Washer_Interface_Ctrl."Init Com Port", "Error In"=w225) -> ("Error Out"=w222:errorcluster)  [unwired: 9 in, 3 out]
          n99 = case shown="No Error" w222 {
            selector: w222 -> [w232 _]
            tunnel: w223 -> [w228 w239]
            tunnel: "Init Com Port Failure: " -> [_ w238]
            tunnel: [w232 w236] -> w220
            tunnel: w219 -> [_ w236]
            tunnel: [w231 w235] -> w217
            tunnel: [_ w234] -> w215
            tunnel: "Init Com Port " -> [w230 _]
            tunnel: [w229 w234] -> w212
            tunnel: [Washer_Status_Ctrl."No Com" ("Status") Washer_Status_Ctrl."No Conf" ("Status")] -> w211
            frame No Error {
              n100 = global read "Globals HCC.vi" "Color Configured"() -> (w231:u32)
              n101 = call "Com Chan Type Conversion.vi"("Com Chan In"=w228) -> ("Com Text 2"=w227:string)  [unwired: 11 in, 3 out]
              n102 = Concatenate Strings(w230, w227) -> (w229:string)
            }
            frame Error {
              n103 = global read "Globals HCC.vi" "Color Uncofigured"() -> (w235:u32)
              n104 = call "Com Chan Type Conversion.vi"("Com Chan In"=w239) -> ("Com Text 2"=w237:string)  [unwired: 11 in, 3 out]
              n105 = Concatenate Strings(w238, w237) -> (w234:string)
            }
          }
          "Init Com port message" <- w212
          n106 = Bundle By Name(cluster=w218, "Color"=w217, "Status"=w211) -> (w216:T1)
        }
        n107 = Array To Spreadsheet String(array=w196, 3:"" ("format string")) -> (spreadsheet string=w195:string)  [unwired: 1 in]
        n108 = Bundle By Name(cluster=w198, "Row A"=w199) -> (w197:T9)
        n109 = flat-sequence {
          tunnel: w195 -> [w208]
          tunnel: [FALSE ("Visible")] -> w193
          frame #0 {
            n110 = local write "Debug Log"(w208) -> ()
          }
        }
        n111 = property on="Init Com port message" class="Str"("Visible"=w193) -> ()  [unwired: 2 in, 2 out]
        n112 = call <vilib>:"Add State(s) to Queue__jki_lib_state_machine.vi"("State(s) in (\"\")"=w206) -> ("States Out"=w205:string)  [unwired: 14 in]
      }
      frame "UI: Cursor Set" {
        # "Argument"
        # "Set and Unset Cursor Busy.\n(Usage: \"UI: Cursor Set >> Busy|Idle\")"
        n113 = case shown="\"Idle\", Default" w240 {
          tunnel: w242 -> [w247 w249]
          tunnel: [w246 w248] -> w241
          frame "Idle", Default {
            n114 = call <vilib>:"Unset Busy.vi"("error in (no error)"=w247) -> ("error out"=w246:errorcluster)  [unwired: 10 in]
          }
          frame "Busy" {
            n115 = call <vilib>:"Set Busy.vi"("error in (no error)"=w249) -> ("error out"=w248:errorcluster)  [unwired: 9 in, 1 out]
          }
        }
        n116 = call <vilib>:"Add State(s) to Queue__jki_lib_state_machine.vi"("State(s) in (\"\")"=w245) -> ("States Out"=w244:string)  [unwired: 14 in]
      }
      frame "UI: Front Panel State" {
        # "Argument"
        # "Set Front Panel Open or Closed\n(Usage: \"UI: Front Panel State >> Open|Close\")"
        n117 = Unbundle By Name(w252) -> ("Core.Current VI Reference"=w251:refnum<vi>)
        n118 = case shown="\"Open\", Default" w250 {
          tunnel: w254 -> [w260 w273]
          tunnel: [w262 w274] -> w253
          tunnel: w251 -> [w261 w271]
          frame "Open", Default {
            n119 = property class="VI"(reference=w261, error in=w260) -> (reference out=w258:refnum<vi>, error out=w259:errorcluster, "Front Panel.Open"=w257:bool)
            n120 = case shown="False" w257 {
              tunnel: [w265 w268] -> w262
              tunnel: w259 -> [w264 w268]
              tunnel: w258 -> [w263 _]
              frame False {
                n121 = invoke class="VI" method="FP.Open"(reference=w263, error in=w264, "Activate"=TRUE, "State"=T8."Standard") -> (error out=w265:errorcluster)  [unwired: 1 in, 4 out]
              }
              frame True {
              }
            }
          }
          frame "Close" {
            n122 = property class="VI"(reference=w271, error in=w273) -> (reference out=w270:refnum<vi>, error out=w272:errorcluster, "Front Panel.Open"=w269:bool)
            n123 = case shown="True" w269 {
              tunnel: [w275 w278] -> w274
              tunnel: w272 -> [w275 w277]
              tunnel: w270 -> [_ w276]
              frame False {
              }
              frame True {
                n124 = invoke class="VI" method="FP.Close"(reference=w276, error in=w277) -> (error out=w278:errorcluster)  [unwired: 1 in, 2 out]
              }
            }
          }
        }
        n125 = call <vilib>:"Add State(s) to Queue__jki_lib_state_machine.vi"("State(s) in (\"\")"=w256) -> ("States Out"=w255:string)  [unwired: 14 in]
      }
      frame "---------- Macro ----------" {
        # "Do not put any code in this frame.\n(It is a separator no-op. You can make a copy of this frame to create a new Macro frame)"
        n126 = call <vilib>:"Add State(s) to Queue__jki_lib_state_machine.vi"("State(s) in (\"\")"=w282) -> ("States Out"=w281:string)  [unwired: 14 in]
      }
      frame "Macro: Initialize" {
        w283 = "Data: Initialize\nInitialize Core Data\nUI: Initialize\nUI: Front Panel State >> Open\nInit Com Ports"  # Data: Initialize Initialize Core Data UI: Initialize UI: Front Panel State >> Open Init Com Ports
        # "Initialization Macro\n(This is called once, when the VI starts)"
        n127 = call <vilib>:"Add State(s) to Queue__jki_lib_state_machine.vi"("State(s) in Front (\"\")"=w283, "State(s) in (\"\")"=w287) -> ("States Out"=w286:string)  [unwired: 13 in]
      }
      frame "Macro: Exit" {
        # "Exit Macro\n(This is called once, when the VI exits)"
        n128 = Unbundle By Name(w294) -> ("Core.Close Panel on Exit?"=w293:bool)
        n129 = Select(t="UI: Front Panel State >> Close", s=w293, f="") -> (s? t:f=w290:string)
        n130 = call <vilib>:"Add State(s) to Queue__jki_lib_state_machine.vi"("State(s) in (\"\")"=w290, "State(s) at Back (\"\")"="Data: Cleanup\nExit") -> ("States Out"=w288:string)  [unwired: 13 in]
        n131 = call <vilib>:"Add State(s) to Queue__jki_lib_state_machine.vi"("State(s) in Front (\"\")"=w288, "State(s) in (\"\")"=w297) -> ("States Out"=w296:string)  [unwired: 13 in]
      }
      frame "---------- New Category ----------" {
        # "Template Separator\n(You can make a copy of, or modify, this frame)"
        n132 = call <vilib>:"Add State(s) to Queue__jki_lib_state_machine.vi"("State(s) in (\"\")"=w301) -> ("States Out"=w300:string)  [unwired: 14 in]
      }
      frame "Read" {
        # "read the serial ports"
        n133 = Unbundle By Name(w310) -> ("Com Array"=w311:u8[], "Row A"=w303:T1[])
        n134 = flat-sequence {
          tunnel: [w316] -> w304
          frame #0 {
            n135 = local read "Partial Messages Out"() -> (w316:cluster{"Partial Message Out":u8[]}[])
            n136 = local write "Reading"(TRUE ("Reading")) -> ()
          }
        }
        n137 = call "Read All Washers.vi"("Com Array"=w311, "HCC  Array In"=w303, "Partial Message Array"=w304) -> ("Log Coms Array"=→"Log Coms Array":string[], "HCC  Array Out"=w302:T1[], "Data Present"=→"Data Present":bool[], "Partial Messages Out"=→"Partial Messages Out":cluster{"Partial Message Out":u8[]}[])  [unwired: 8 in, 1 out]
        n138 = flat-sequence {
          tunnel: w302 -> [w318]
          frame #0 {
            n139 = local write "Row A"(w318) -> ()
            "Reading" <- FALSE ("Reading")
          }
        }
        n140 = Bundle By Name(cluster=w310, "Row A"=w302) -> (w309:T9)
        n141 = local write "Row C"(w302) -> ()
        n142 = local write "Row B"(w302) -> ()
        n143 = local write "Row D"(w302) -> ()
        n144 = local write "Row E"(w302) -> ()
        n145 = local write "Row F"(w302) -> ()
        n146 = call <vilib>:"Add State(s) to Queue__jki_lib_state_machine.vi"("State(s) in Front (\"\")"="Add Select Data" ("State(s) in Front (\"\")"), "State(s) in (\"\")"=w314) -> ("States Out"=w313:string)  [unwired: 13 in]
      }
      frame "Add Select Data" {
        # "Your code here.\n(You can make a copy of, or modify, this frame)"
        n147 = Unbundle By Name(w328) -> ("Label Com Array"=w327:string[][], "Row A"=w326:T1[])
        n148 = for {
          tunnel: w327 -> [w346] mode=indexing
          tunnel: w326 -> [w341] mode=indexing
          tunnel: [w340] -> w325
          tunnel: [w340] -> w322
          stop <- w342 stop-if-true
          n149 = Unbundle By Name(w341) -> ("Debug Log"=w340:string)
          n150 = Index Array(array=w346, index=0) -> (element=w343:string)
          n151 = Equal?(x=w343, y="Select Station") -> (x = y?=w342:bool)
        }
        n152 = global read "Globals HCC.vi" "Max Length of Display Data"() -> (w319:i32)
        n153 = String Length(string=w322) -> (length=w321:i32)
        n154 = Greater Than 0?(x=w321) -> (x > 0?=w320:bool)
        n155 = case shown="True" w320 {
          tunnel: w325 -> [_ w336]
          tunnel: "Debug Log" -> [w334 w335]
          tunnel: [w334 w338] -> w323
          tunnel: w319 -> [_ w337]
          frame False {
          }
          frame True {
            n156 = Concatenate Strings(w336, w335) -> (w339:string)
            n157 = String Subset(string=w339, length (rest)=w337) -> (substring=w338:string)  [unwired: 1 in]
          }
        }
        n158 = flat-sequence {
          tunnel: w323 -> [w333]
          frame #0 {
            n159 = local write "Debug Log"(w333) -> ()
            n160 = property on="Debug Log" class="Str"("Text.Scroll Position"=u32 100000) -> ()  [unwired: 2 in, 2 out]
          }
        }
        n161 = call <vilib>:"Add State(s) to Queue__jki_lib_state_machine.vi"("State(s) in (\"\")"=w331) -> ("States Out"=w330:string)  [unwired: 14 in]
      }
      frame "Write" {
        # "Robocopy every hour"
        # "Do not put any code in this frame.\n(It is a separator no-op. You can make a copy of this frame to create a new UI frame)"
        n162 = local read "FileVersionInfo Out"() -> (w351:T5)
        n163 = Unbundle By Name(w367) -> ("Save File Directory"=w355:path, "Library Batch File"=w356:path, "Row A"=w353:T1[], "Last Hour"=w354:string, "Data Set ID"=w352:string)
        n164 = Unbundle By Name(w351) -> ("ProductName"=w348:string, "FileVersion"=w347:string)
        n165 = Format Date/Time String(time format string (%c)="%H") -> (date/time string=w361:string)  [unwired: 2 out]
        n166 = Equal?(x=w354, y=w361) -> (x = y?=w364:bool)
        n167 = local read "Current Filename"() -> (w359:path)
        n168 = Build Array(w348, w347) -> (w350:string[])
        n169 = Build Array(w350) -> (w349:string[][])
        n170 = Not(x=w364) -> (.not. x?=w363:bool)
        n171 = call "File Washer HCC.vi"("Washer Array"=w353, "Dryer s,h Data Dir"=w355, "Header"=w349, "Data Set ID"=w352, "Last Save Hour"=w354, "error in (no error)"=w358, "Sample Data Current Filename"=w359) -> ("Last Save Hour Out"=w360:string, "Sample Data Current Filename Out"=w362:path, "error out"=w357:errorcluster)  [unwired: 5 in, 1 out]
        "Current Filename" <- w362
        n172 = case shown="True" w363 {
          tunnel: w362 -> [_ _]
          tunnel: w356 -> [_ w373]
          tunnel: w355 -> [_ _]
          frame False {
          }
          frame True {
            w370 = "\"" ("string")
            n173 = Path To String(path=w373) -> (string=w372:string)
            n174 = Concatenate Strings(w370, w372, w370) -> (w371:string)
            n175 = call <vilib>:"System Exec.vi"("run minimized? (F)"=TRUE, "command line"=w371) -> ("error out"=→"Saving":errorcluster)  [unwired: 6 in, 3 out]
          }
        }
        n176 = Bundle By Name(cluster=w367, "Last Hour"=w360) -> (w366:T9)
        n177 = call <vilib>:"Add State(s) to Queue__jki_lib_state_machine.vi"("State(s) in (\"\")"=w369) -> ("States Out"=w368:string)  [unwired: 14 in]
      }
      frame "Enable Log" {
        # "send the enable log command to all of the stations in err."
        n178 = Unbundle By Name(w378) -> ("Com Array"=w377:u8[], "Row A"=w376:T1[])
        n179 = for {
          tunnel: w376 -> [w389] mode=indexing
          tunnel: w377 -> [w386] mode=indexing
          tunnel: w380 -> [w385]
          tunnel: [w384] -> w379
          n180 = Unbundle By Name(w389) -> ("Status"=w388:T2)
          n181 = Equal?(x=w388, y=Washer_Status_Ctrl."Err" ("Status")) -> (x = y?=w387:bool)
          n182 = case shown="True" w387 {
            tunnel: w386 -> [_ w393]
            tunnel: w385 -> [w390 w392]
            tunnel: [w390 w391] -> w384
            frame False {
            }
            frame True {
              w398 = u8 28 items=["CMD_Entry_Command", "CMD_Load_Control", "RQST_Input_Status", "CMD_LED_Control", "RQST_Encoder_Position_Status", "RQST_A2D_Status", "RQST_Switch_States_Status", "CMD_Buzzer_Control", "CMD_Shift_to_Spin", "CMD_Shift_to_Agitate", "RQST_Mode_Shift_Complete_Status", "CMD_Control_Inverter", "CMD_Spin_Action", "CMD_Agitate_Action", "RQST_Total_Switch_Status", "RQST_Total_Encoder_Status", "CMD_Test_Eeprom", "RQST_Eeprom_Test_Status", "CMD_Power_Mode", "RQST_Error_Status", "RQST_Get_Version", "CMD_Set_Personality", "RQST_Get_Personality", "CMD_Serial_Number", "RQST_Serial_Number_Status", "CMD_Model_Number", "RQST_Model_Number_Status", "CMD_Enter_Boot_Loader", "CMD_Enable_Debug_Log"] ("Command")
              w395 = u8 255  # Tester Source Address
              w394 = u8 35  # Washer Destination Address
              n183 = call "Com Chan Type Conversion.vi"("Com Chan"=w393) -> ("VISA resource name"=w396:refnum<visa-resource-name>)  [unwired: 11 in, 3 out]
              n184 = call "GEA2_ICP_Washer_SM.vi"("ComPort"=w396, "Destination Address"=w394, "Source Address"=w395, "Mode"=GEA2_Washer_Interface_Ctrl."SendCMD", "Byte Data"=u8[] [1], "Error In"=w392, "Command"=w398) -> ("Error Out"=w391:errorcluster)  [unwired: 5 in, 3 out]
            }
          }
        }
        n185 = call <vilib>:"Add State(s) to Queue__jki_lib_state_machine.vi"("State(s) in (\"\")"=w382) -> ("States Out"=w381:string)  [unwired: 14 in]
      }
    }
    n186 = Equal To 0?(x=w3) -> (x = 0?=w4:bool)
    n187 = call "Build String Array w Max Size.vi"("Initialize"=w4, "string"=w6) -> ("Array"=→"Debug State Array":string[])  [unwired: 9 in]
  }
